vi "Assert Contains.vi"(7 "Label":string="Assert Contains", 8 "error in (no error)":errorcluster, 10 "Array":string[](array[string]), 11 "Item":string) -> (0 "error out":errorcluster)   [LabVIEW 2017, in "Assert Extensions.lvclass"]
uses:
  Assert Extensions.lvclass
  <vilib>/addons/_JKI Toolkits/Caraya/classes/Properties.Assert/Properties.Assert.lvclass
  C:/Program Files/National Instruments/LabVIEW 2017/vi.lib/addons/_JKI Toolkits/Caraya/classes/Properties/Properties.lvclass
  <vilib>/addons/_JKI Toolkits/Caraya/classes/Assert/Assert.lvclass
  <vilib>/addons/_JKI Toolkits/Caraya/classes/Properties/Properties.lvclass
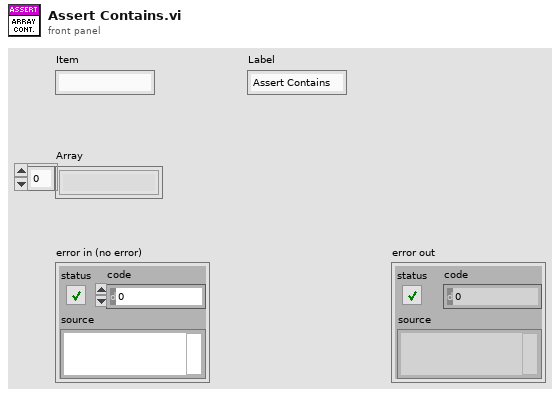
[diagram p1: front panel]
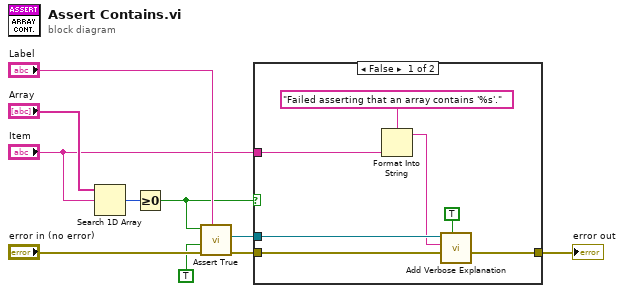
[diagram p0: block diagram]
diagram:
  n1 = Search 1D Array(1D array="Array", element="Item") -> (index of element=w8:i32)  [unwired: 1 in]
  n2 = Greater Or Equal To 0?(x=w8) -> (x >= 0?=w3:bool)
  n3 = call <vilib>:"Assert True.vi"("Label"="Label", "error in (no error)"="error in (no error)", "Register with caller test (F)"=TRUE, "True?"=w3) -> ("error out"=w5:errorcluster, "Properties"=w2:refnum<class "Properties.Assert.lvclass">)  [unwired: 6 in]
  n4 = case shown="False" w3 {
    tunnel: w5 -> [w16 w18]
    tunnel: [w15 w18] -> w4
    tunnel: w2 -> [w14 _]
    tunnel: "Item" -> [w13 _]
    frame False {
      n5 = Format Into String(format string="Failed asserting that an array contains '%s'.", w13) -> (resulting string=w11:string)  [unwired: 2 in, 1 out]
      n6 = call <vilib>:"Add Verbose Explanation.vi"("overwrite?"=TRUE, "error in (no error)"=w16, "Verbose Explanation"=w11, "Properties"=w14) -> ("error out"=w15:errorcluster)  [unwired: 6 in, 1 out]
    }
    frame True {
    }
  }
  "error out" <- w4
